vi "dropDownMenu.vi"() -> ()   [LabVIEW 2020]
panel:
  in  "CLOSE SHOP, BANG GANG":bool
  in  "Menu: You Hungry?":T1(ring)
  out "Cost and Reply":string
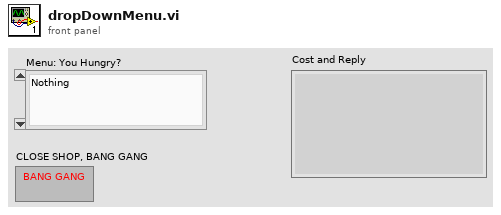
[diagram p1: front panel]
types:
  T1 = enum16{"Nothing", "Beer", "Char Kway teow", "Bak Chor Mee", ""}
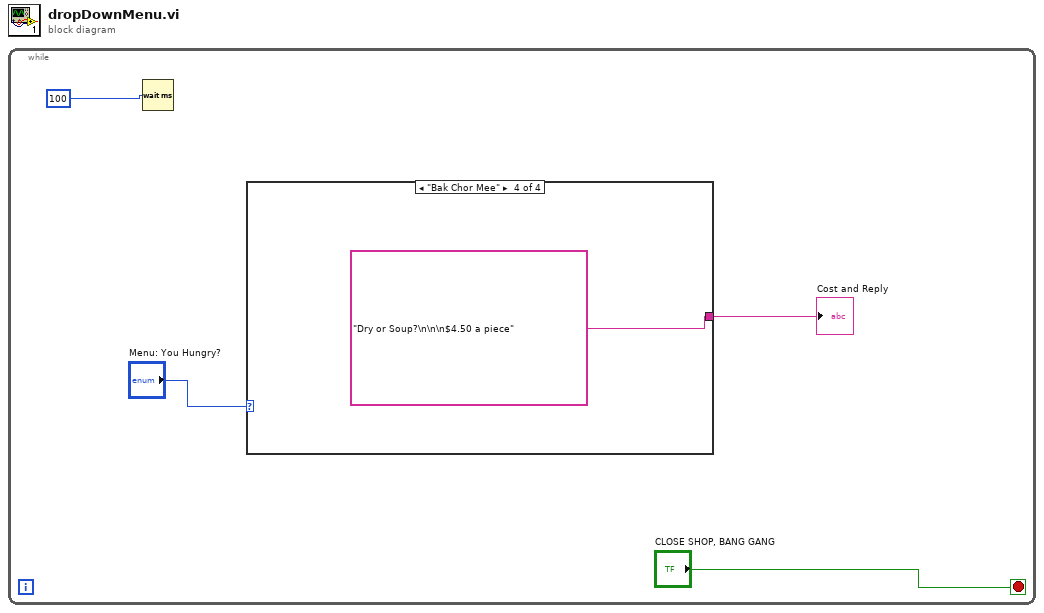
[diagram p0: block diagram]
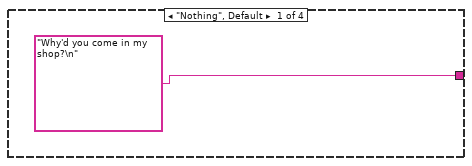
[diagram p2: hidden frame]
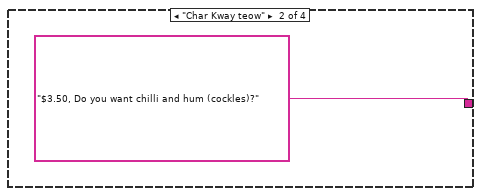
[diagram p3: hidden frame]
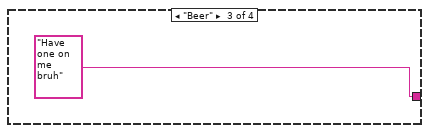
[diagram p4: hidden frame]
diagram:
  n1 = while {
    stop <- "CLOSE SHOP, BANG GANG" stop-if-true
    n2 = Wait (ms)(milliseconds to wait=100) -> ()  [unwired: 1 out]
    n3 = case shown="\"Bak Chor Mee\"" "Menu: You Hungry?" {
      tunnel: ["Why'd you come in my shop?\n" "$3.50, Do you want chilli and hum (cockles)?" "Have one on me bruh" "Dry or Soup?\n\n\n$4.50 a piece"] -> w4
      frame "Nothing", Default {
      }
      frame "Char Kway teow" {
      }
      frame "Beer" {
      }
      frame "Bak Chor Mee" {
      }
    }
    "Cost and Reply" <- w4
  }
